vi "K_grating.vi"(2 "error in (no error)":errorcluster, 3 "Grating, gr/mm 2":T1) -> (0 "error out":errorcluster, 1 "K_grating":i16)   [LabVIEW 2017, in "Monochromator.lvlib" / "PTI.lvlib"]
doc: "grating gr conversion to number"
uses:
  PTI.lvlib
  Controls/GratingValues.ctl
  Monochromator.lvlib
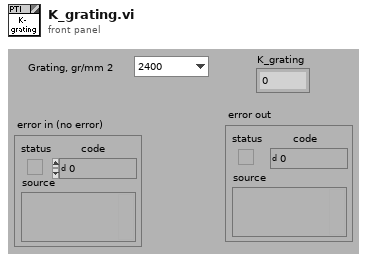
[diagram p1: front panel]
types:
  T1 = typedef "Monochromator.lvlib/GratingValues.ctl" = enum16{"2400", "1800", "1200", "600", "300", "150"}
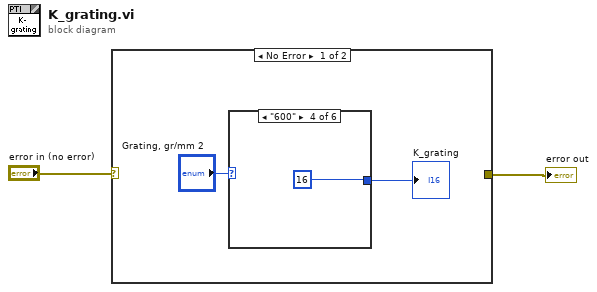
[diagram p0: block diagram]
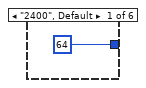
[diagram p2: hidden frame]
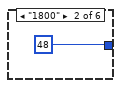
[diagram p3: hidden frame]
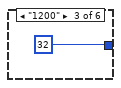
[diagram p4: hidden frame]
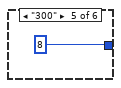
[diagram p5: hidden frame]
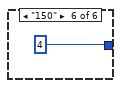
[diagram p6: hidden frame]
diagram:
  n1 = case shown="No Error" "error in (no error)" {
    selector: "error in (no error)" -> [_ w11]
    tunnel: [_ w11] -> w2
    frame No Error {
      n2 = case shown="\"600\"" "Grating, gr/mm 2" {
        tunnel: [64 48 32 16 8 4] -> w4
        frame "2400", Default {
        }
        frame "1800" {
        }
        frame "1200" {
        }
        frame "600" {
        }
        frame "300" {
        }
        frame "150" {
        }
      }
      "K_grating" <- w4
    }
    frame Error {
    }
  }
  "error out" <- w2
